vi "SVFA Wrap or Unwrap Phase.vi"   [LabVIEW 2017]
doc: "Wraps the phase spectra to the specified range, so that all phase values are coerced to the specified band. You also can use this VI to unwrap phase spectra to eliminate discontinuities with absolute values exceeding 180 degrees = pi radians = 0.5 cycles. Wire data to the <B>phase spectrum in</B> input to determine the polymorphic instance to use or manually select the instance."
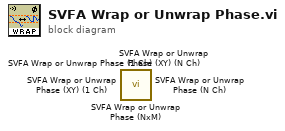
[diagram p0: block diagram]
diagram:
  n1 = call <vilib>:"SVFA Wrap or Unwrap Phase (NxM).vi"() -> ()  [unwired: 16 in, 4 out]
  n2 = call <vilib>:"SVFA Wrap or Unwrap Phase (XY) (N Ch).vi"() -> ()  [unwired: 16 in, 4 out]
  n3 = call <vilib>:"SVFA Wrap or Unwrap Phase (XY) (1 Ch).vi"() -> ()  [unwired: 16 in, 4 out]
  n4 = call <vilib>:"SVFA Wrap or Unwrap Phase (N Ch).vi"() -> ()  [unwired: 16 in, 4 out]
  n5 = call <vilib>:"SVFA Wrap or Unwrap Phase (1 Ch).vi"() -> ()  [unwired: 16 in, 4 out]
